vi "close target with engines.vi"(6 "timeout (-1)":i32=-1, 8 "error in":errorcluster, 10 "Engine Runtime Interfaces":refnum<class "Engine Runtime Interface.lvclass">[](array[class]), 11 "Target Runtime":refnum<class "PL_Target Runtime.lvclass">) -> (0 "error out":errorcluster)   [LabVIEW 2013, in "PL_Target Runtime.lvclass"]
doc: "Closes the references to both a Target and an array of Engines running on that target."
uses:
  PL_Target Runtime.lvclass
  <vilib>/NI/Module Execution Interface/Engine Runtime/Engine Runtime Interface.lvclass
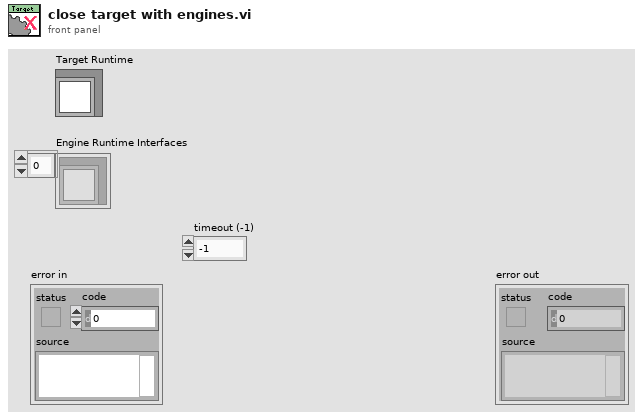
[diagram p1: front panel]
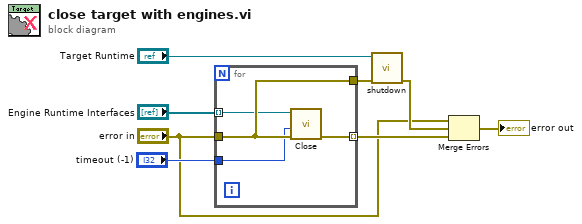
[diagram p0: block diagram]
diagram:
  n1 = for {
    tunnel: "error in" -> [w11]
    tunnel: [w12] -> w4 mode=indexing
    tunnel: [w11] -> w8
    tunnel: "Engine Runtime Interfaces" -> [w10] mode=indexing
    tunnel: "timeout (-1)" -> [w9]
    n2 = call-dynamic "Close.vi"("error in"=w11, "timeout (-1)"=w9, "Engine Runtime Interface in"=w10) -> ("error out"=w12:errorcluster)  [unwired: 8 in]
  }
  n3 = call-dynamic "shutdown.vi"("error in"=w8, "Target Runtime in"="Target Runtime") -> ("error out"=w5:errorcluster)  [unwired: 9 in]
  n4 = Merge Errors("error in", w5, w4) -> (→"error out":errorcluster)
